vi "EPS-Initialize.vi"(8 "error in":errorcluster, 11 "EPS Setting In":T1) -> (0 "error out":errorcluster, 3 "EPS Setting Out":T1)   [LabVIEW 2018]
uses:
  Data Def/EPS-Setting.ctl
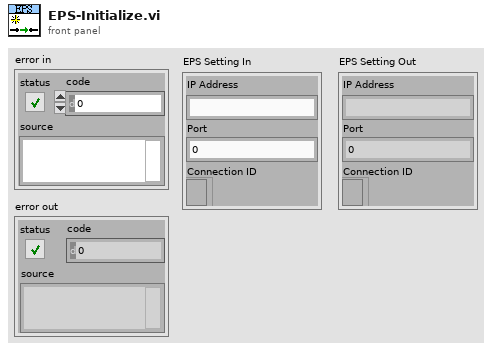
[diagram p1: front panel]
types:
  T1 = typedef "EPS-Setting.ctl" = cluster{"IP Address":string, "Port":u16, "Connection ID":refnum<k5>}
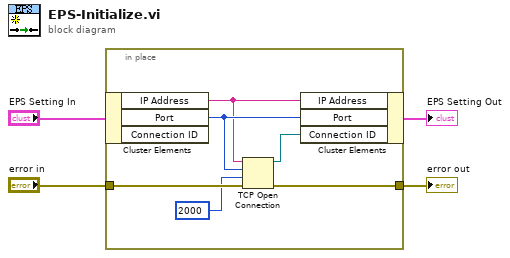
[diagram p0: block diagram]
diagram:
  n1 = in-place {
    in-place-border: "error in" -> [w10]
    in-place-border: [w9] -> w3
    n2 = in-place-cluster #1("EPS Setting In") -> ("IP Address"=w5:string, "Port"=w6:u16)  [unwired: 1 out]
    n3 = TCP Open Connection(address=w5, remote port or service name=w6, timeout ms (60000)=2000, error in (no error)=w10) -> (connection ID=w7:refnum<k5>, error out=w9:errorcluster)  [unwired: 1 in]
    n4 = in-place-cluster #1("IP Address"=w5, "Port"=w6, "Connection ID"=w7) -> (→"EPS Setting Out":T1)
  }
  "error out" <- w3
